vi "Get Formatting Settings - Bookmark Options.vi"(8 "error in (no error)":errorcluster {"code" format="Error %.0f"}, 11 "VIDoc Printer In":refnum<class "VIDoc Printer.lvclass">) -> (0 "error out":errorcluster {"code" format="Error %.0f"}, 2 "Bookmark Descriptions":T1={"Bookmarks as New Line in VI Descriptions"=TRUE, "Unique Bookmark Tags Only"=TRUE, "Include Tag and Text"=TRUE}, 3 "VIDoc Printer Out":refnum<class "VIDoc Printer.lvclass">)   [LabVIEW 2023, in "VIDoc Printer.lvlib" / "VIDoc Printer.lvclass"]
uses:
  VIDoc Printer.lvclass
  Settings/Printer Settings/Bookmark Options.ctl
  VIDoc Printer.lvclass/VIDoc Printer.ctl
  Settings/Printer Settings/Printer Settings.lvclass
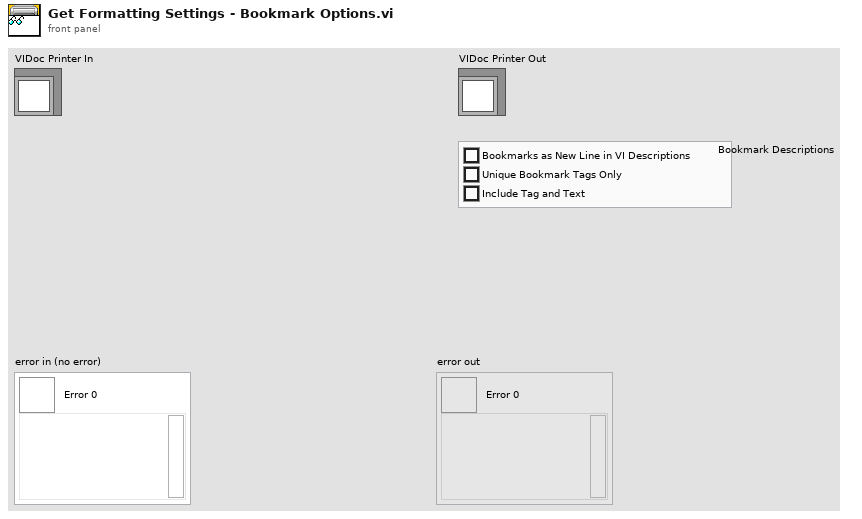
[diagram p1: front panel]
types:
  T1 = typedef "VIDoc Printer.lvlib/Printer Settings.lvclass/Bookmark Options.ctl" = cluster{"Bookmarks as New Line in VI Descriptions":bool, "Unique Bookmark Tags Only":bool, "Include Tag and Text":bool}
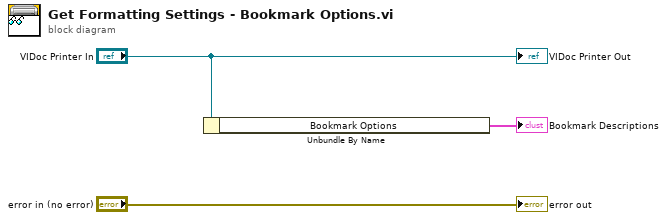
[diagram p0: block diagram]
diagram:
  n1 = Unbundle By Name("VIDoc Printer In") -> ("Bookmark Options"=→"Bookmark Descriptions":T1)
  "error out" <- "error in (no error)"
  "VIDoc Printer Out" <- "VIDoc Printer In"
